vi "LJUD U3RAW Feedback.vi"(7 "Comm Settings":T1={"Open LabJack "=TRUE, "Address"="1", "FirstFound"=TRUE}, 8 "error in (no error)":errorcluster, 9 "# Data Bytes to Read":i32=2, 10 "Data":u8[](array[numeric])=[1, 0, 31] format="%.0x", 11 "Handle In":i32) -> (0 "error out":errorcluster, 2 "Data Read":u8[](array[numeric]) format="%.0x", 3 "Handle Out":i32)   [LabVIEW 2021]
panel:
  out "Read":u8[](array[numeric]) format="%.0x"
  # "Chcksm8"
  # "F8"
  # "#DataWords"
  # "0x00"
  # "Chcksm16"
  # "Chcksm16"
  # "Error"
  # "Error Seq"
  # "Echo Byte"
  # "Data0"
  # "If open is false,\nthen a valid\nhandle must be\npassed in."
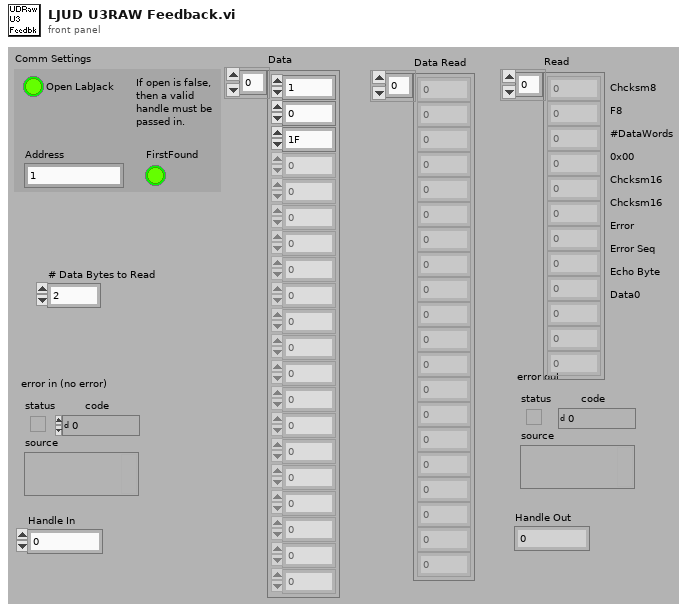
[diagram p1: front panel]
types:
  T1 = cluster{"Open LabJack ":bool, "Address":string, "FirstFound":bool}
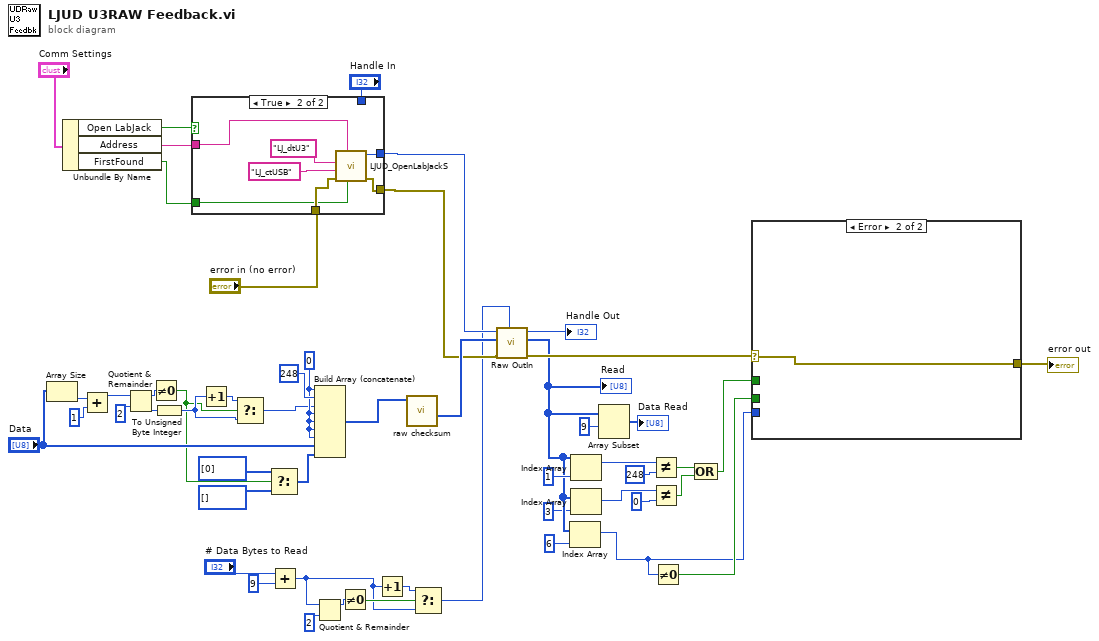
[diagram p0: block diagram]
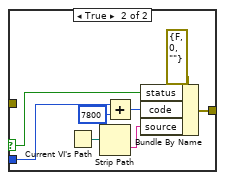
[diagram p3: hidden frame]
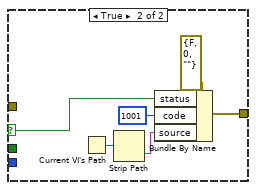
[diagram p4: hidden frame]
diagram:
  w26 = u8 0 ("Input Element")
  n1 = Array Size(array="Data") -> (size(s)=w20:i32)
  n2 = Unbundle By Name("Comm Settings") -> ("Open LabJack"=w43:bool, "Address"=w42:string, "FirstFound"=w41:bool)
  n3 = Add(x=w20, y=u8 1) -> (x+y=w19:i32)
  n4 = Quotient & Remainder(x=w19, y=2) -> (x-y*floor(x/y)=w24:i32, floor(x/y)=w18:i32)
  n5 = Not Equal To 0?(x=w24) -> (x != 0?=w15:bool)
  n6 = To Unsigned Byte Integer(number=w18) -> (unsigned 8bit integer=w17:u8)
  n7 = case shown="True" w43 {
    tunnel: w42 -> [_ w58]
    tunnel: "error in (no error)" -> [w54 w59]
    tunnel: [w54 w60] -> w46
    tunnel: [w53 w61] -> w45
    tunnel: w41 -> [_ w57]
    tunnel: "Handle In" -> [w53 _]
    frame False {
    }
    frame True {
      n8 = call "LJUD_OpenLabJackS.vi"("FirstFound"=w57, "Address"=w58, "error in"=w59, "ConnectionType"="LJ_ctUSB", "DeviceType"="LJ_dtU3") -> ("error out"=w60:errorcluster, "Handle"=w61:i32)  [unwired: 4 in, 1 out]
    }
  }
  n9 = Increment(x=w17) -> (x+1=w16:u8)
  n10 = Select(t=w16, s=w15, f=w17) -> (s? t:f=w14:u8)
  n11 = Select(t=u8[] [0] ("Input Array"), s=w15, f=u8[] [] ("Input Array")) -> (s? t:f=w23:u8[])
  n12 = Add(x="# Data Bytes to Read", y=9) -> (x+y=w9:i32)
  n13 = Build Array (concatenate)(w26, u8 248 ("Input Element"), w14, w26, w26, w26, w26, "Data", w23) -> (w51:u8[])
  n14 = Quotient & Remainder(x=w9, y=2) -> (x-y*floor(x/y)=w12:i32)  [unwired: 1 out]
  n15 = Not Equal To 0?(x=w12) -> (x != 0?=w10:bool)
  n16 = Increment(x=w9) -> (x+1=w11:i32)
  n17 = call "raw checksum.vi"("Array"=w51) -> ("Array Output"=w49:u8[])  [unwired: 3 in, 7 out]
  n18 = Select(t=w11, s=w10, f=w9) -> (s? t:f=w8:i32)
  n19 = call "Raw OutIn.vi"("# of bytes to read in"=w8, "error in"=w46, "Raw Out"=w49, "Handle In"=w45) -> ("error out"=w36:errorcluster, "Raw In"=w5:u8[], "Handle Out"=→"Handle Out":i32)  [unwired: 4 in, 1 out]
  "Read" <- w5
  n20 = Index Array(array=w5, index=6 ("Index")) -> (element=w2:u8)
  n21 = Index Array(array=w5, index=1 ("Index")) -> (element=w3:u8)
  n22 = Index Array(array=w5, index=3 ("Index")) -> (element=w1:u8)
  n23 = Array Subset(array=w5, index=9 ("Array Index")) -> (→"Data Read":u8[])  [unwired: 1 in]
  n24 = Not Equal?(x=w3, y=u8 248 ("Input Element")) -> (x != y?=w38:bool)
  n25 = Not Equal?(x=w1, y=u8 0 ("Input Element")) -> (x != y?=w37:bool)
  n26 = Not Equal To 0?(x=w2) -> (x != 0?=w34:bool)
  n27 = Compound Arithmetic op=OR(w38, w37) -> (w35:bool)
  n28 = case shown="Error" w36 {
    selector: w36 -> [w62 w86]
    tunnel: w35 -> [w66 _]
    tunnel: w34 -> [w65 _]
    tunnel: w2 -> [w64 _]
    tunnel: [w63 w86] -> w33
    frame No Error {
      n29 = case shown="False" w66 {
        selector: w66 -> [_ w80]
        tunnel: w65 -> [w70 _]
        tunnel: w64 -> [w69 _]
        tunnel: [w68 w82] -> w63
        tunnel: w62 -> [w67 _]
        frame False {
          n30 = case shown="False" w70 {
            selector: w70 -> [_ w73]
            tunnel: w69 -> [_ w74]
            tunnel: [w71 w72] -> w68
            tunnel: w67 -> [w71 _]
            frame False {
            }
            frame True {
              n31 = Current VI's Path() -> (path=w77:path)
              n32 = Strip Path(path=w77) -> (name=w76:string)  [unwired: 1 out]
              n33 = Add(x=w74, y=7800) -> (x+y=w78:i32)
              n34 = Bundle By Name(cluster=errorcluster {"status"=FALSE, "code"=0, "source"=""} ("error IO"), "status"=w73, "code"=w78, "source"=w76) -> (w72:errorcluster)
            }
          }
        }
        frame True {
          n35 = Current VI's Path() -> (path=w85:path)
          n36 = Strip Path(path=w85) -> (name=w84:string)  [unwired: 1 out]
          n37 = Bundle By Name(cluster=errorcluster {"status"=FALSE, "code"=0, "source"=""} ("error IO"), "status"=w80, "code"=1001, "source"=w84) -> (w82:errorcluster)
        }
      }
    }
    frame Error {
    }
  }
  "error out" <- w33
